vi "Set DisplayCtr Color.vi"(8 "error in (no error)":errorcluster, 9 "Mode":enum16{"Label", "Caption", "Text"}(ring), 10 "Color Box":u32(colorbox), 11 "Ctr Ref":refnum<vi>) -> (0 "error IO":errorcluster)   [LabVIEW 2014]
panel:
  out "Ctr Ref out":refnum<vi>
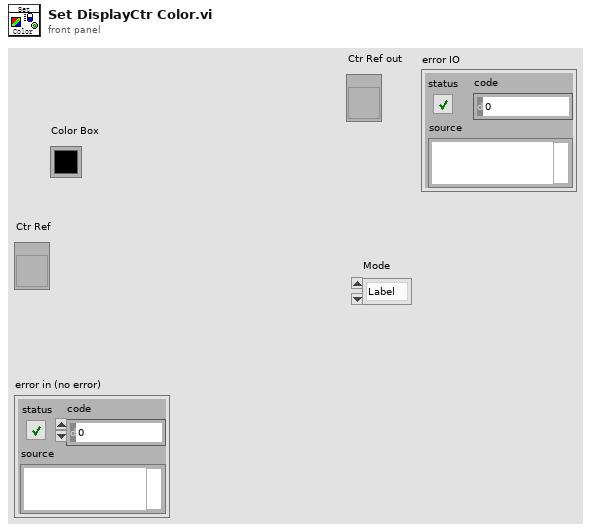
[diagram p1: front panel]
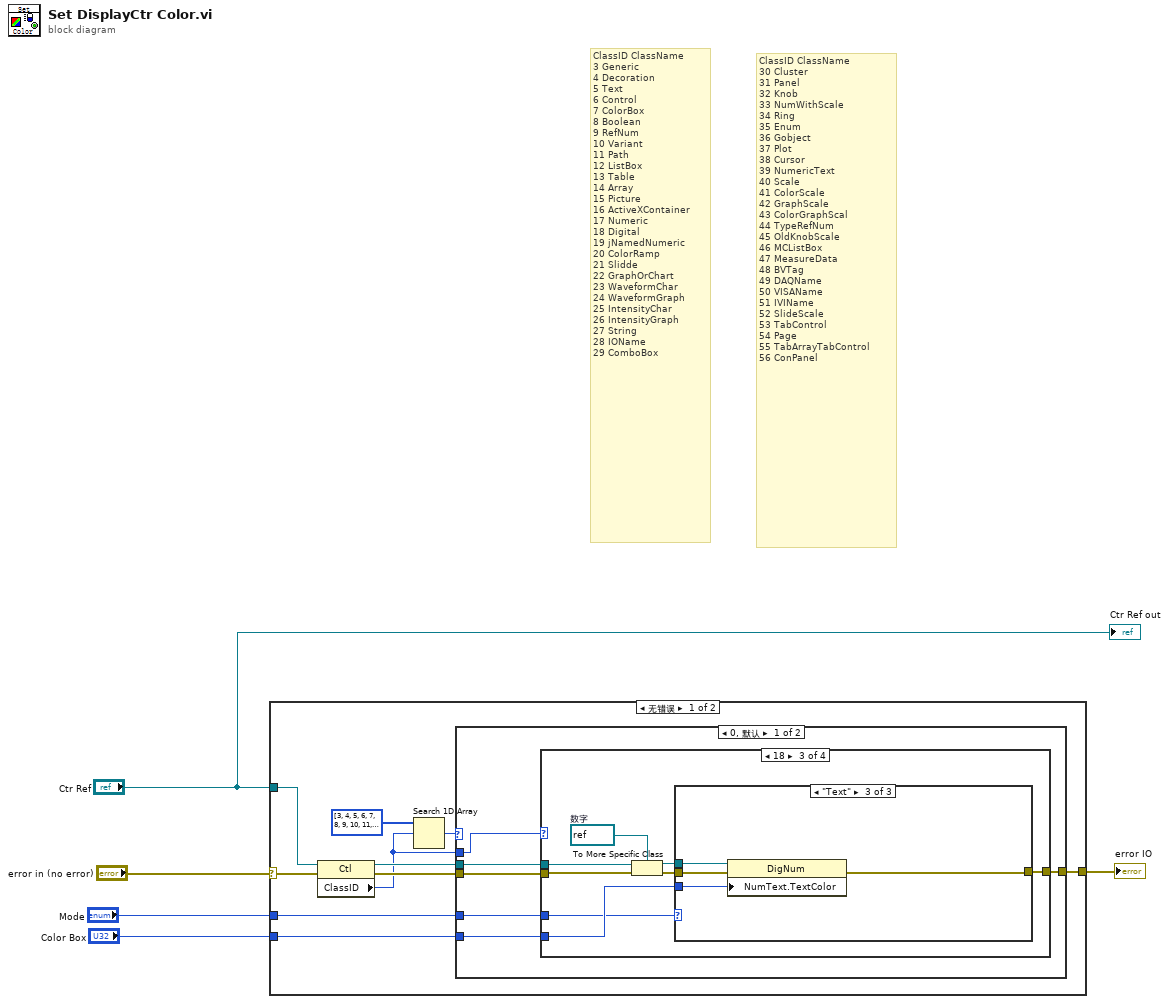
[diagram p0: block diagram]
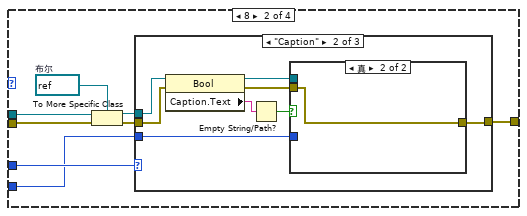
[diagram p3: hidden frame]
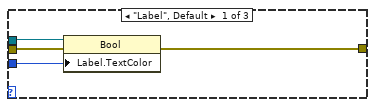
[diagram p4: hidden frame]
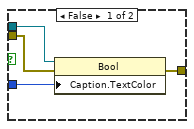
[diagram p5: hidden frame]
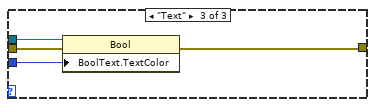
[diagram p6: hidden frame]
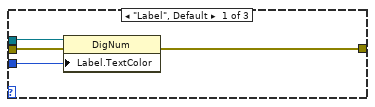
[diagram p7: hidden frame]
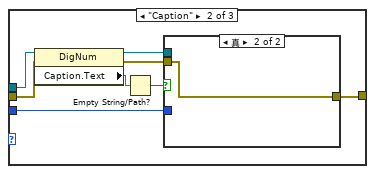
[diagram p8: hidden frame]
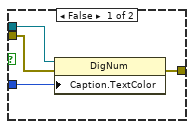
[diagram p9: hidden frame]
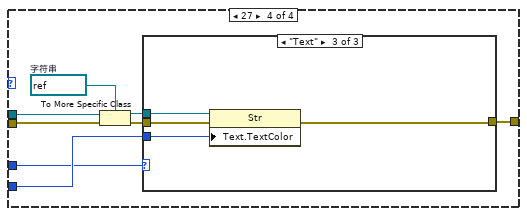
[diagram p10: hidden frame]
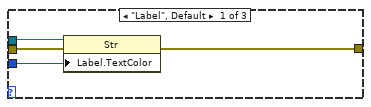
[diagram p11: hidden frame]
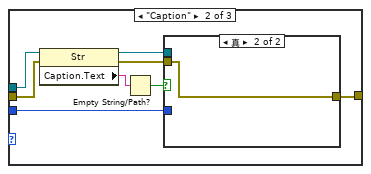
[diagram p12: hidden frame]
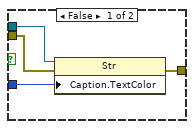
[diagram p13: hidden frame]
diagram:
  # "ClassID\tClassName\n30\tCluster\n31\tPanel\n32\tKnob\n33\tNumWithScale\n34\tRing\n35\tEnum\n36\tGobject\n37\tPlot\n38\tCursor\n39\tNumericText\n40\tScale\n41\tColorScale\n42\tGraphScale\n43\tColorGraphScal\n44\tTypeRefNum\n45\tOldKnobScale\n46\tMCListBox\n47\tMeasureData\n48\tBVTag\n49\tDAQName\n50\tVISAName\n51\tIVIName\n52\tSlideScale\n53\tTabControl\n54\tPage\n55\tTabArrayTabControl\n56\tConPanel"
  # "ClassID\tClassName\n3\tGeneric\n4\tDecoration\n5\tText\n6\tControl\n7\tColorBox\n8\tBoolean\n9\tRefNum\n10\tVariant\n11\tPath\n12\tListBox\n13\tTable\n14\tArray\n15\tPicture\n16\tActiveXContainer\n17\tNumeric\n18\tDigital\n19\tjNamedNumeric\n20\tColorRamp\n21\tSlidde\n22\tGraphOrChart\n23\tWaveformChar\n24\tWaveformGraph\n25\tIntensityChar\n26\tIntensityGraph\n27\tString\n28\tIOName\n29\tComboBox"
  n1 = case shown="无错误" "error in (no error)" {
    selector: "error in (no error)" -> [w15 w111]
    tunnel: "Ctr Ref" -> [w14 _]
    tunnel: "Mode" -> [w9 _]
    tunnel: "Color Box" -> [w8 _]
    tunnel: [w7 w111] -> w1
    frame No Error {
      n2 = property class="Ctl"(reference=w14, error in=w15) -> (reference out=w11:refnum<vi>, error out=w10:errorcluster, "ClassID"=w6:u32)
      n3 = Search 1D Array(1D array=u32[] [3, 4, 5, 6, 7, 8, 9, 10, 11, 12, 13, 14, 15, 16, 17, 18, 19, 20, 21, 22, 23, 24, 25, 26, 27, 28, 29, 30, 31, 32, 33, 34, 35, 36, 37, 38, 39, 40, 41, 42, 43, 44, 45, 46, 47, 48, 49, 50, 51, 52, 53, 54, 55, 56] ("Array"), element=w6) -> (index of element=w12:i32)  [unwired: 1 in]
      n4 = case shown="0, 默认" w12 {
        tunnel: w11 -> [w20 _]
        tunnel: w10 -> [w21 w110]
        tunnel: w9 -> [w19 _]
        tunnel: w8 -> [w18 _]
        tunnel: [w17 w110] -> w7
        tunnel: w6 -> [w16 _]
        frame 0, Default {
          n5 = case shown="18" w16 {
            tunnel: w21 -> [w22 w30 w54 w84]
            tunnel: w20 -> [_ w29 w53 w83]
            tunnel: w19 -> [_ w25 w55 w81]
            tunnel: w18 -> [_ w24 w56 w82]
            tunnel: [w22 w23 w52 w85] -> w17
            frame 0, Default {
            }
            frame 8 {
              w28 = refnum<vi> refnum  # 布尔
              n6 = To More Specific Class(target class=w28, reference=w29, error in=w30) -> (specific class reference=w26:refnum<vi>, error out=w27:errorcluster)
              n7 = case shown="\"Caption\"" w25 {
                tunnel: w27 -> [w34 w39 w51]
                tunnel: w26 -> [w33 w40 w50]
                tunnel: w24 -> [w32 w42 w49]
                tunnel: [w31 w41 w48] -> w23
                frame "Label", Default {
                  n8 = property class="Bool"(reference=w33, error in=w34, "Label.TextColor"=w32) -> (error out=w31:errorcluster)  [unwired: 1 out]
                }
                frame "Caption" {
                  n9 = property class="Bool"(reference=w40, error in=w39) -> (reference out=w36:refnum<vi>, error out=w35:errorcluster, "Caption.Text"=w38:string)
                  n10 = Empty String/Path?(string/path=w38) -> (empty?=w37:bool)
                  n11 = case shown="真" w37 {
                    tunnel: w42 -> [w46 _]
                    tunnel: [w45 w47] -> w41
                    tunnel: w36 -> [w44 _]
                    tunnel: w35 -> [w43 w47]
                    frame False {
                      n12 = property class="Bool"(reference=w44, error in=w43, "Caption.TextColor"=w46) -> (error out=w45:errorcluster)  [unwired: 1 out]
                    }
                    frame True {
                    }
                  }
                }
                frame "Text" {
                  n13 = property class="Bool"(reference=w50, error in=w51, "BoolText.TextColor"=w49) -> (error out=w48:errorcluster)  [unwired: 1 out]
                }
              }
            }
            frame 18 {
              w59 = refnum<vi> refnum  # 数字
              n14 = To More Specific Class(target class=w59, reference=w53, error in=w54) -> (specific class reference=w57:refnum<vi>, error out=w58:errorcluster)
              n15 = case shown="\"Text\"" w55 {
                tunnel: w58 -> [w63 w68 w80]
                tunnel: w57 -> [w62 w69 w79]
                tunnel: w56 -> [w61 w71 w78]
                tunnel: [w60 w70 w77] -> w52
                frame "Label", Default {
                  n16 = property class="DigNum"(reference=w62, error in=w63, "Label.TextColor"=w61) -> (error out=w60:errorcluster)  [unwired: 1 out]
                }
                frame "Caption" {
                  n17 = property class="DigNum"(reference=w69, error in=w68) -> (reference out=w65:refnum<vi>, error out=w64:errorcluster, "Caption.Text"=w67:string)
                  n18 = Empty String/Path?(string/path=w67) -> (empty?=w66:bool)
                  n19 = case shown="真" w66 {
                    tunnel: w71 -> [w75 _]
                    tunnel: [w74 w76] -> w70
                    tunnel: w65 -> [w73 _]
                    tunnel: w64 -> [w72 w76]
                    frame False {
                      n20 = property class="DigNum"(reference=w73, error in=w72, "Caption.TextColor"=w75) -> (error out=w74:errorcluster)  [unwired: 1 out]
                    }
                    frame True {
                    }
                  }
                }
                frame "Text" {
                  n21 = property class="DigNum"(reference=w79, error in=w80, "NumText.TextColor"=w78) -> (error out=w77:errorcluster)  [unwired: 1 out]
                }
              }
            }
            frame 27 {
              w88 = refnum<vi> refnum  # 字符串
              n22 = To More Specific Class(target class=w88, reference=w83, error in=w84) -> (specific class reference=w86:refnum<vi>, error out=w87:errorcluster)
              n23 = case shown="\"Text\"" w81 {
                tunnel: w87 -> [w92 w97 w109]
                tunnel: w86 -> [w91 w98 w108]
                tunnel: w82 -> [w90 w100 w107]
                tunnel: [w89 w99 w106] -> w85
                frame "Label", Default {
                  n24 = property class="Str"(reference=w91, error in=w92, "Label.TextColor"=w90) -> (error out=w89:errorcluster)  [unwired: 1 out]
                }
                frame "Caption" {
                  n25 = property class="Str"(reference=w98, error in=w97) -> (reference out=w94:refnum<vi>, error out=w93:errorcluster, "Caption.Text"=w96:string)
                  n26 = Empty String/Path?(string/path=w96) -> (empty?=w95:bool)
                  n27 = case shown="真" w95 {
                    tunnel: w100 -> [w104 _]
                    tunnel: [w103 w105] -> w99
                    tunnel: w94 -> [w102 _]
                    tunnel: w93 -> [w101 w105]
                    frame False {
                      n28 = property class="Str"(reference=w102, error in=w101, "Caption.TextColor"=w104) -> (error out=w103:errorcluster)  [unwired: 1 out]
                    }
                    frame True {
                    }
                  }
                }
                frame "Text" {
                  n29 = property class="Str"(reference=w108, error in=w109, "Text.TextColor"=w107) -> (error out=w106:errorcluster)  [unwired: 1 out]
                }
              }
            }
          }
        }
        frame -1 {
        }
      }
    }
    frame Error {
    }
  }
  "error IO" <- w1
  "Ctr Ref out" <- "Ctr Ref"
